vi "Delete Install Files Missing From Source.vi"(8 "Error In":errorcluster, 11 "Configuration":T1) -> (0 "Error Out":errorcluster, 2 "Deleted From Souce":path[](array[path]), 3 "Configuration":T1)   [LabVIEW 2011, in "LVH-Build-Tools.lvlib"]
uses:
  LVH-Build-Tools.lvlib
  Type Defs/Configuration.ctl
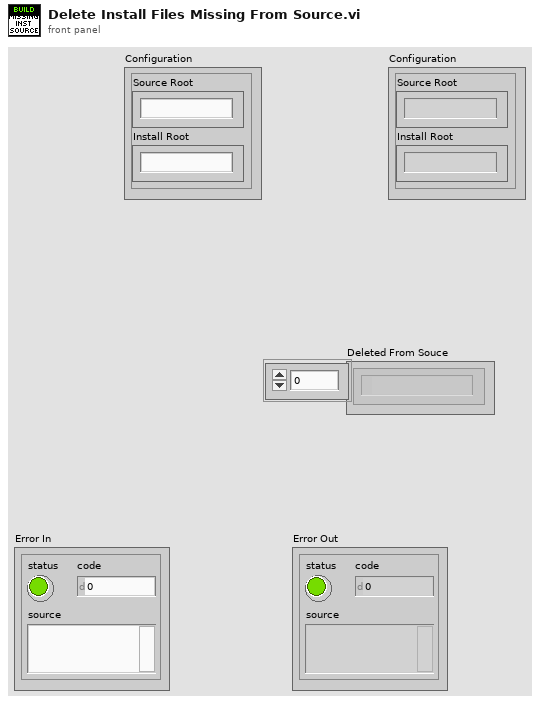
[diagram p1: front panel]
types:
  T1 = typedef "LVH-Build-Tools.lvlib/Configuration.ctl" = cluster{"Source Root":string, "Install Root":string, "Components":string[], "Ignore":string[]}
  T2 = enum16{"Left Button", "Center Button", "Right Button", "Window Close"}
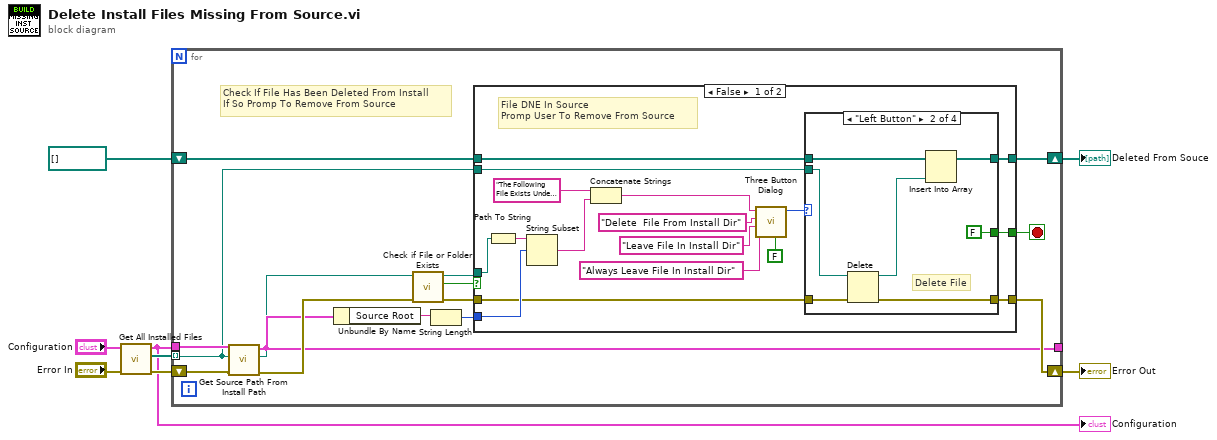
[diagram p0: block diagram]
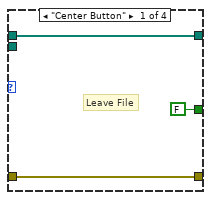
[diagram p2: hidden frame]
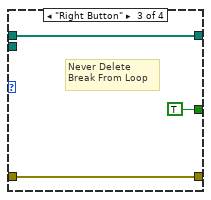
[diagram p3: hidden frame]
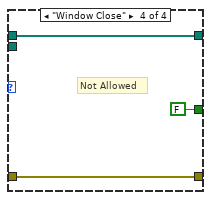
[diagram p4: hidden frame]
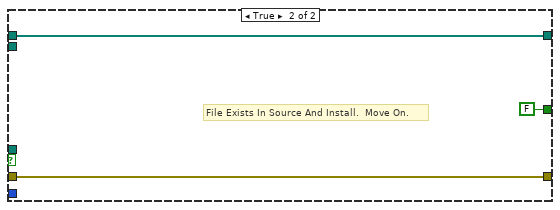
[diagram p5: hidden frame]
diagram:
  n1 = call "Get All Installed Files.vi"("Error In"="Error In", "Configuration"="Configuration") -> ("Error Out"=w4:errorcluster, "All Installed Files"=w5:path[], "Configuration"=w1:T1)  [unwired: 7 in]
  "Configuration" <- w1
  n2 = for {
    tunnel: w5 -> [w10] mode=indexing
    shift-right: [w20] -> w8
    shift-left: w4 -> [w17]
    tunnel: [w15] -> _
    shift-right: [w18] -> w7
    shift-left: path[] [] ("Array in") -> [w19]
    tunnel: w1 -> [w11]
    stop <- w9 stop-if-true
    # "Check If File Has Been Deleted From Install \nIf So Promp To Remove From Source"
    n3 = call "Get Source Path From Install Path.vi"("Error In"=w17, "Install File Path"=w10, "Configuration"=w11) -> ("Error Out"=w16:errorcluster, "Install File Path"=w12:path, "Configuraiton"=w15:T1)  [unwired: 5 in, 1 out]
    n4 = Unbundle By Name(w15) -> ("Source Root"=w14:string)
    n5 = call <vilib>:"Check if File or Folder Exists.vi"("error in (no error)"=w16, "path"=w12) -> ("error out"=w22:errorcluster, "file or folder exists?"=w23:bool, "dup path"=w13:path)  [unwired: 7 in]
    n6 = String Length(string=w14) -> (length=w21:i32)
    n7 = case shown="False" w23 {
      tunnel: w22 -> [w36 w59]
      tunnel: w21 -> [w40 _]
      tunnel: [w35 w59] -> w20
      tunnel: w19 -> [w34 w58]
      tunnel: [w33 w58] -> w18
      tunnel: w10 -> [w31 _]
      tunnel: w13 -> [w30 _]
      tunnel: [w24 FALSE] -> w9
      frame False {
        # "File DNE In Source\nPromp User To Remove From Source"
        n8 = Path To String(path=w30) -> (string=w32:string)
        n9 = String Subset(string=w32, offset (0)=w40) -> (substring=w39:string)  [unwired: 1 in]
        n10 = Concatenate Strings("The Following File Exists Under The Install Directory But Not The Source Directory.  If you choose not to delete this file it will be synced with the source directory next time you run Sync Source.vi\n\n", w39) -> (w38:string)
        n11 = call <vilib>:"Three Button Dialog.vi"("Allow user to close window? (TRUE)"=FALSE, "Right Button Text (\"Cancel\")"="Always Leave File In Install Dir" ("F button name (\"Cancel\")"), "Center Button Text (\"No\")"="Leave File In Install Dir" ("F button name (\"Cancel\")"), "Left Button Text (\"Yes\")"="Delete  File From Install Dir" ("T button name (\"OK\")"), "message"=w38) -> ("Which Button?"=w37:T2)  [unwired: 6 in]
        n12 = case shown="\"Left Button\"" w37 {
          tunnel: w36 -> [w43 w50 w51 w54]
          tunnel: [w43 w49 w51 w54] -> w35
          tunnel: w34 -> [w42 w48 w52 w56]
          tunnel: [w42 w46 w52 w56] -> w33
          tunnel: w31 -> [_ w45 _ _]
          tunnel: [FALSE FALSE TRUE FALSE] -> w24
          frame "Center Button" {
            # "Leave File"
          }
          frame "Left Button" {
            # "Delete File"
            n13 = Delete(path (use dialog)=w45, error in=w50) -> (deleted path=w47:path, error out=w49:errorcluster)  [unwired: 3 in, 1 out]
            n14 = Insert Into Array(array=w48, new element=w47) -> (w46:path[])  [unwired: 1 in]
          }
          frame "Right Button" {
            # "Never Delete\nBreak From Loop"
          }
          frame "Window Close" {
            # "Not Allowed"
          }
        }
      }
      frame True {
        # "File Exists In Source And Install.  Move On."
      }
    }
  }
  "Error Out" <- w8
  "Deleted From Souce" <- w7
